vi "Command Drive To Cube With Heading.vi"(8 "Timeout":dbl=3.5, 9 "Heading":dbl, 10 "Speed":dbl=0.45, 11 "Startup":bool) -> (0 "Right Wheel":dbl, 1 "Reinit":bool, 2 "Left Wheel":dbl, 3 "Completed":bool)   [LabVIEW 2017]
uses:
  Utility VIs/Refnum Names.vi
  Drive/Drive Globals.vi
  Intake/Intake Globals.vi
panel:
  in  "Turn Gain":dbl=-0.06
  # "Alpha .06"
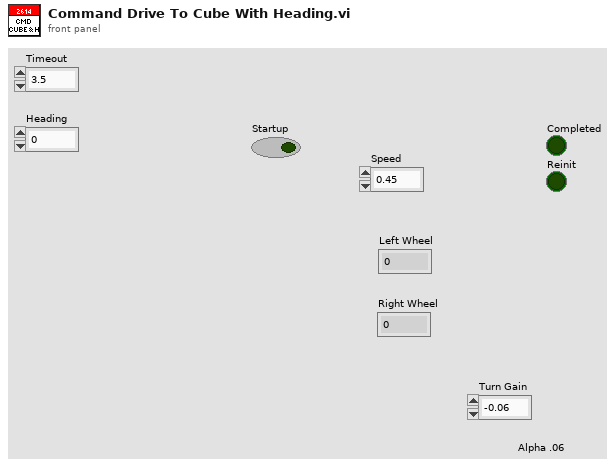
[diagram p1: front panel]
types:
  T1 = typedef "WPI_MotorControlDeviceRef.ctl" = cluster{"DeviceStatus":errorcluster, "Type":T2, "PWM":cluster{"PWM Channel":T3, "DeadBand":T4}, "CAN":cluster{"Device Number":u8, "SetOutput VI Ref":variant, "GetOutput VI Ref":variant, "Enable VI Ref":variant, "Disable VI Ref":variant, "Data":variant}, "Invert":bool, "DIO PWM":cluster{"PWM \"Enable\" Channel":T3, "DIOChannel":T5, "PWM Rate":dbl}}
  T2 = typedef "WPI_MotorControlType.ctl" = enum16{"PWM", "CAN", "DIO PWM"}
  T3 = typedef "FPGA_DIOPWMChannel.ctl" = enum8{"PWM 0", "PWM 1", "PWM 2", "PWM 3", "PWM 4", "PWM 5", "PWM 6", "PWM 7", "PWM 8", "PWM 9", "PWM MXP 0", "PWM MXP 1", "PWM MXP 2", "PWM MXP 3", "PWM MXP 4", "PWM MXP 5", "PWM MXP 6", "PWM MXP 7", "PWM MXP 8", "PWM MXP 9", "Invalid"}
  T4 = typedef "WPI_PWMDeadband.ctl" = cluster{"Name":string, "maxPositivePwm":i32, "minPositivePwm":i32, "centerPwm":i32, "maxNegativePwm":i32, "minNegativePwm":i32, "angularRange":u16}
  T5 = typedef "FPGA_DIOChannel.ctl" = enum8{"DIO 0", "DIO 1", "DIO 2", "DIO 3", "DIO 4", "DIO 5", "DIO 6", "DIO 7", "DIO 8", "DIO 9", "DIO MXP 0", "DIO MXP 1", "DIO MXP 2", "DIO MXP 3", "DIO MXP 4", "DIO MXP 5", "DIO MXP 6", "DIO MXP 7", "DIO MXP 8", "DIO MXP 9", "DIO MXP 10", "DIO MXP 11", "DIO MXP 12", "DIO MXP 13", "DIO MXP 14", "DIO MXP 15", "SPI Port CS1", "SPI Port CS2", "SPI Port CS3", "SPI Port MISO", "SPI Port MOSI", "Invalid"}
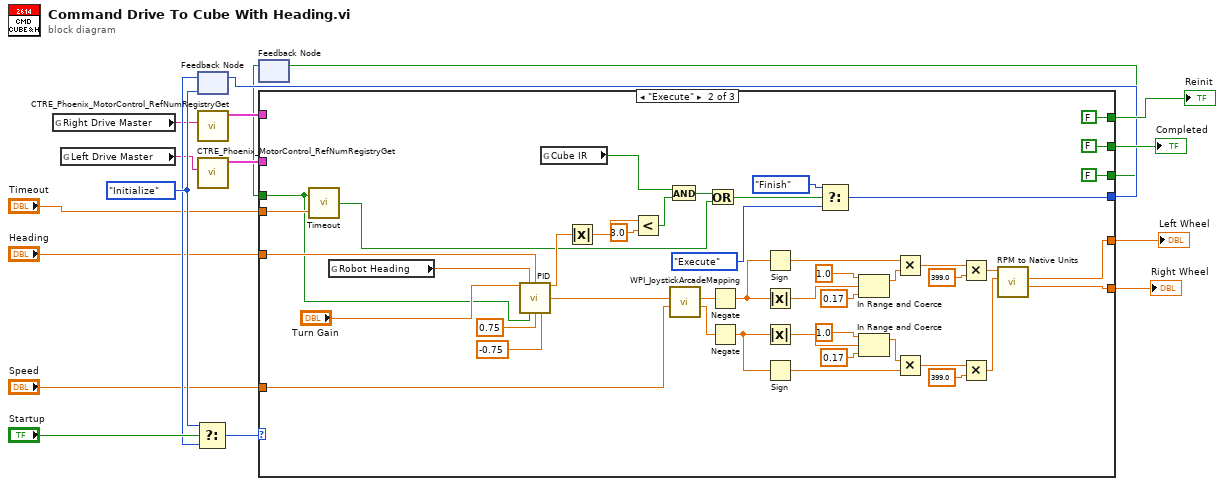
[diagram p0: block diagram]
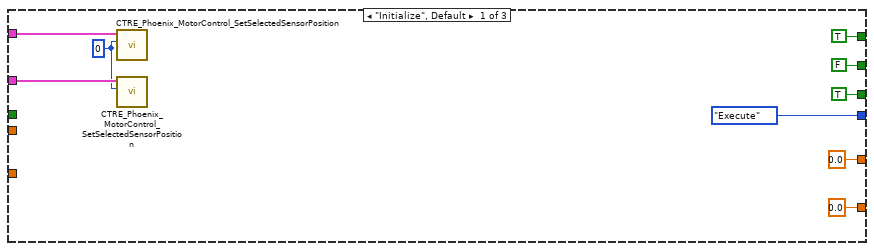
[diagram p2: hidden frame]
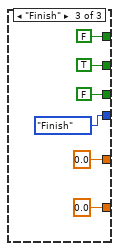
[diagram p3: hidden frame]
diagram:
  w16 = enum16{"Initialize", "Execute", "Finish"}."Initialize"
  n1 = global read "Refnum Names.vi" "Right Drive Master"() -> (w7:string)
  n2 = global read "Refnum Names.vi" "Left Drive Master"() -> (w8:string)
  n3 = feedback #1(w16) -> (w12:enum16{"Initialize", "Execute", "Finish"})
  n4 = Select(t=w16, s="Startup", f=w12) -> (s? t:f=w17:enum16{"Initialize", "Execute", "Finish"})
  n5 = call <vilib>:"CTRE_Phoenix_MotorControl_RefNumRegistryGet.vi"("refnum name"=w7) -> ("PhoenixMotorControlDevRef"=w6:T1)  [unwired: 9 in, 1 out]
  n6 = call <vilib>:"CTRE_Phoenix_MotorControl_RefNumRegistryGet.vi"("refnum name"=w8) -> ("PhoenixMotorControlDevRef"=w5:T1)  [unwired: 9 in, 1 out]
  n7 = feedback #2() -> (w2:bool)  [unwired: 1 in]
  n8 = case shown="\"Execute\"" w17 {
    tunnel: [FALSE FALSE TRUE] -> w15
    tunnel: [TRUE FALSE FALSE] -> w14
    tunnel: [enum16{"Initialize", "Execute", "Finish"}."Execute" w69 enum16{"Initialize", "Execute", "Finish"}."Finish"] -> w13
    tunnel: "Speed" -> [_ w30 _]
    tunnel: [0.0 ("Left Wheel Velocity") w33 0.0] -> w10
    tunnel: [0.0 ("Right Wheel Velocity") w32 0.0] -> w9
    tunnel: w6 -> [w21 _ _]
    tunnel: w5 -> [w22 _ _]
    tunnel: "Heading" -> [_ w59 _]
    tunnel: [TRUE FALSE FALSE] -> w3
    tunnel: w2 -> [_ w28 _]
    tunnel: "Timeout" -> [_ w52 _]
    frame "Initialize", Default {
      w20 = 0
      n9 = call <vilib>:"CTRE_Phoenix_MotorControl_SetSelectedSensorPosition.vi"("New Sensor Position"=w20, "PhoenixMotorControlDevRef"=w21) -> ()  [unwired: 8 in, 2 out]
      n10 = call <vilib>:"CTRE_Phoenix_MotorControl_SetSelectedSensorPosition.vi"("New Sensor Position"=w20, "PhoenixMotorControlDevRef"=w22) -> ()  [unwired: 8 in, 2 out]
    }
    frame "Execute" {
      n11 = call "Timeout.vi"("Timeout"=w52, "Initialize"=w28) -> ("Timed Out?"=w50:bool)
      n12 = global read "Drive Globals.vi" "Robot Heading"() -> (w31:dbl)
      n13 = call "PID.vi"("Kp"="Turn Gain", "Process Variable"=w31, "Goal"=w59, "Reinit"=w28, "Max Ouput"=0.75, "Min Output"=-0.75) -> ("Current Error"=w60:dbl, "Command"=w58:dbl)  [unwired: 7 in, 1 out]
      n14 = global read "Intake Globals.vi" "Cube IR"() -> (w29:bool)
      n15 = Absolute Value(x=w60) -> (abs(x)=w62:dbl)
      n16 = Less?(x=w62, y=3.0) -> (x < y?=w61:bool)
      n17 = And(x=w29, y=w61) -> (x .and. y?=w64:bool)
      n18 = call <vilib>:"WPI_JoystickArcadeMapping.vi"("Y axis value"=w30, "X axis value"=w58) -> ("Right Motor Value"=w56:dbl, "Left Motor Value"=w57:dbl)  [unwired: 8 in]
      n19 = Or(x=w64, y=w50) -> (x .or. y?=w51:bool)
      n20 = Negate(x=w57) -> (-x=w46:dbl)
      n21 = Negate(x=w56) -> (-x=w47:dbl)
      n22 = Sign(1:w46) -> (0:w45:dbl)
      n23 = Absolute Value(x=w46) -> (abs(x)=w49:dbl)
      n24 = Absolute Value(x=w47) -> (abs(x)=w48:dbl)
      n25 = Sign(1:w47) -> (0:w40:dbl)
      n26 = Select(t=enum16{"Initialize", "Execute", "Finish"}."Finish", s=w51, f=enum16{"Initialize", "Execute", "Finish"}."Execute") -> (s? t:f=w69:enum16{"Initialize", "Execute", "Finish"})
      n27 = In Range and Coerce(upper limit=1.0, x=w49, lower limit=0.17) -> (coerced(x)=w44:dbl)  [unwired: 1 out]
      n28 = In Range and Coerce(upper limit=1.0, x=w48, lower limit=0.17) -> (coerced(x)=w41:dbl)  [unwired: 1 out]
      n29 = Multiply(x=w45, y=w44) -> (x*y=w43:dbl)
      n30 = Multiply(x=w41, y=w40) -> (x*y=w42:dbl)
      n31 = Multiply(x=w43, y=399.0) -> (x*y=w35:dbl)
      n32 = Multiply(x=w42, y=399.0) -> (x*y=w34:dbl)
      n33 = call "RPM to Native Units.vi"("Right RPM"=w34, "Left RPM"=w35) -> ("Right Out"=w32:dbl, "Left Out"=w33:dbl)  [unwired: 6 in, 1 out]
    }
    frame "Finish" {
    }
  }
  "Completed" <- w15
  "Reinit" <- w14
  "Left Wheel" <- w10
  "Right Wheel" <- w9
  n34 = feedback-in #1(w13) -> ()
  n35 = feedback-in #2(w3) -> ()
